vi "LDA_Spectra_slow.vi"() -> (5 "Plug in titles":string[](array[string]), 7 "Plug in values":string[](array[string]))   [LabVIEW 2010]
uses:
  Globals/Plug_in_data_global.vi
  Globals/LDA_meas_global_1.vi
  Globals/Meas_global.vi
  <vilib>/gmath/NI_Gmath.lvlib
panel:
  out "Power Spectrum FFT {X} Frequency":dbl[](array[numeric]) format="%.2f"
  out "XY Graph":T1(graph)
  # "You must have just these two indicators on the connector pane of the vi"
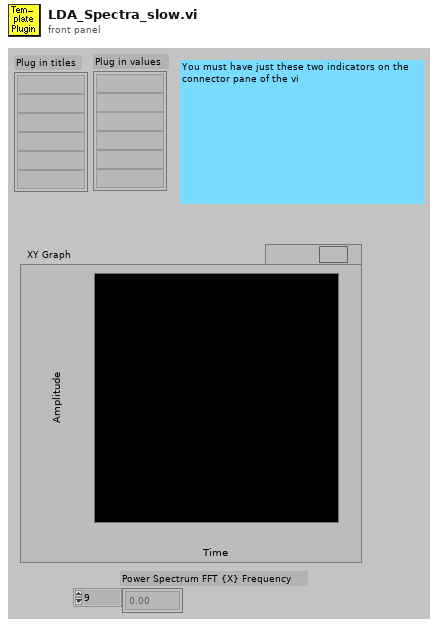
[diagram p1: front panel]
types:
  T1 = cluster{"Power Spectrum FFT {X} Frequency":dbl[], "Power Spectrum FFT {X}":dbl[]}
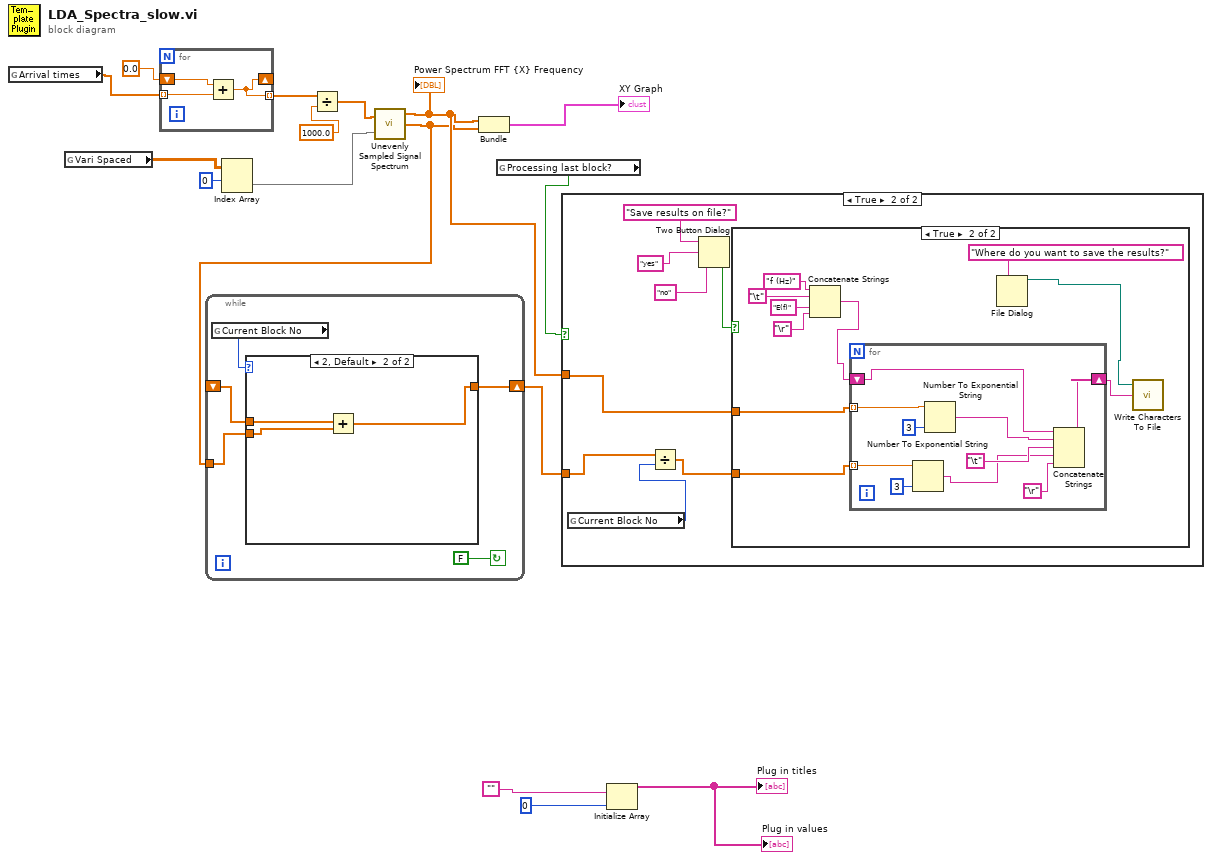
[diagram p0: block diagram]
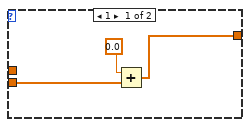
[diagram p2: hidden frame]
diagram:
  n1 = global read "LDA_meas_global_1.vi" "Arrival times"() -> (w10:dbl[])
  n2 = global read "Plug_in_data_global.vi" "Vari Spaced"() -> (w13:dbl[][])
  n3 = for {
    shift-right: [w17] -> _
    shift-left: 0.0 -> [w19]
    tunnel: w10 -> [w18] mode=indexing
    tunnel: [w17] -> w8 mode=indexing
    n4 = Add(x=w19, y=w18) -> (x+y=w17:dbl)
  }
  n5 = Index Array(array=w13, index (row)=0) -> (element=w2:dbl[])  [unwired: 1 in]
  n6 = Divide(x=w8, y=1000.0) -> (x/y=w1:dbl[])
  n7 = call <vilib>:"Unevenly Sampled Signal Spectrum.vi"("XTime"=w1, "X"=w2) -> ("Power Spectrum FFT {X} Frequency"=w4:dbl[], "Power Spectrum FFT {X}"=w3:dbl[])  [unwired: 1 out]
  "Power Spectrum FFT {X} Frequency" <- w4
  n8 = while {
    tunnel: w3 -> [w21]
    shift-right: [w20] -> w6
    shift-left: _ -> [w22]
    stop <- FALSE continue-if-true
    n9 = global read "Meas_global.vi" "Current Block No"() -> (w23:i32)
    n10 = case shown="2, Default" w23 {
      tunnel: w22 -> [_ w30]
      tunnel: w21 -> [w26 w29]
      tunnel: [w25 w28] -> w20
      frame 1 {
        n11 = Add(x=0.0, y=w26) -> (x+y=w25:dbl[])
      }
      frame 2, Default {
        n12 = Add(x=w30, y=w29) -> (x+y=w28:dbl[])
      }
    }
  }
  n13 = Bundle("Power Spectrum FFT {X} Frequency"=w4, "Power Spectrum FFT {X}"=w3) -> (→"XY Graph":T1)  [unwired: 1 in]
  n14 = global read "Meas_global.vi" "Processing last block?"() -> (w5:bool)
  n15 = case shown="True" w5 {
    tunnel: w4 -> [_ w32]
    tunnel: w6 -> [_ w34]
    frame False {
    }
    frame True {
      n16 = global read "Meas_global.vi" "Current Block No"() -> (w31:i32)
      n17 = Divide(x=w34, y=w31) -> (x/y=w33:dbl[])
      n18 = Two Button Dialog(message="Save results on file?", 1:"no", 2:"yes") -> (T button?=w35:bool)
      n19 = case shown="True" w35 {
        tunnel: w32 -> [_ w39]
        tunnel: w33 -> [_ w40]
        frame False {
        }
        frame True {
          n20 = Concatenate Strings("f (Hz)", "\t", "E(f)", "\r") -> (w41:string)
          n21 = for {
            shift-right: [w51] -> w47
            shift-left: w41 -> [w52]
            tunnel: w39 -> [w50] mode=indexing
            tunnel: w40 -> [w49] mode=indexing
            n22 = Number To Exponential String(number=w49, precision (6)=i16 3) -> (E-format string=w54:string)  [unwired: 2 in]
            n23 = Number To Exponential String(number=w50, precision (6)=i16 3) -> (E-format string=w57:string)  [unwired: 2 in]
            n24 = Concatenate Strings(w52, w57, "\t", w54, "\r") -> (w51:string)
          }
          n25 = File Dialog(7:"Where do you want to save the results?" ("prompt")) -> (3:w46:path)  [unwired: 6 in, 3 out]
          n26 = call <vilib>:"Write Characters To File.vi"("character string"=w47, "file path (dialog if empty)"=w46) -> ()  [unwired: 3 in, 1 out]
        }
      }
    }
  }
  n27 = Initialize Array("", 0) -> (→"Plug in values" →"Plug in titles":string[])
